vi "setLockin_phi.vi"(8 "error in (no error)":errorcluster, 9 "new phi (deg)":dbl, 10 "lockin Channel":i32, 11 "Channels: Lockin":T1={"REF f (Hz)"=[13.0], "REF phi (deg)"=[0.0]} {"REF phi (deg)" format="%#_3g"}) -> (0 "error out":errorcluster, 3 "Channels: Lockin":T1={"REF f (Hz)"=[13.0], "REF phi (deg)"=[0.0]} {"REF phi (deg)" format="%#_3g"})   [LabVIEW 2016]
uses:
  Typedefs/REF-cluster.ctl
  Typedefs/REF_f-array.ctl
  Typedefs/REF_phi-array.ctl
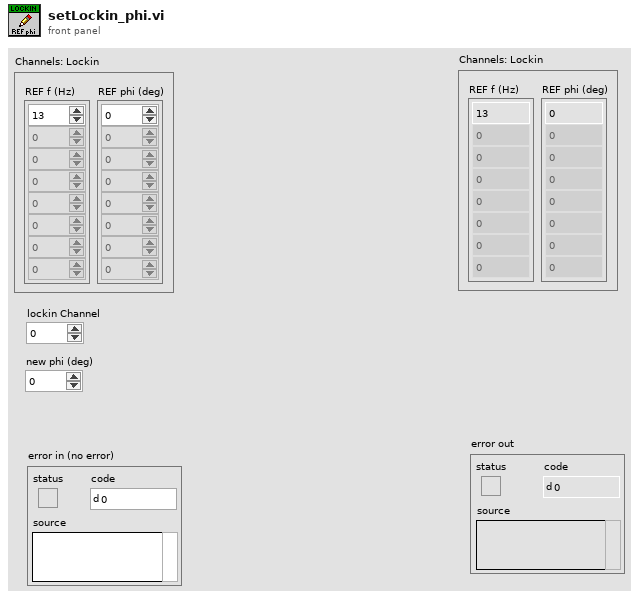
[diagram p1: front panel]
types:
  T1 = typedef "REF-cluster.ctl" = cluster{"REF f (Hz)":T2, "REF phi (deg)":T3}
  T2 = typedef "REF_f-array.ctl" = dbl[]
  T3 = typedef "REF_phi-array.ctl" = dbl[]
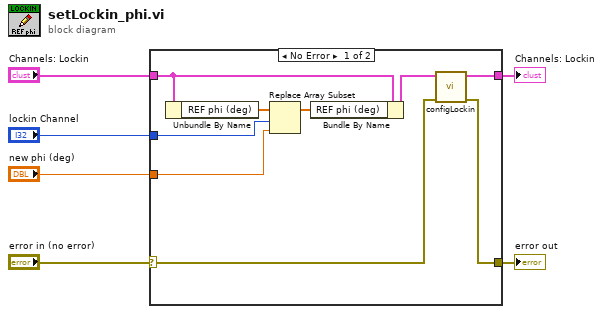
[diagram p0: block diagram]
diagram:
  n1 = case shown="No Error" "error in (no error)" {
    selector: "error in (no error)" -> [w8 w17]
    tunnel: "Channels: Lockin" -> [w13 w16]
    tunnel: [w9 w16] -> w5
    tunnel: "lockin Channel" -> [w12 _]
    tunnel: "new phi (deg)" -> [w11 _]
    tunnel: [w7 w17] -> w1
    frame No Error {
      n2 = Unbundle By Name(w13) -> ("REF phi (deg)"=w14:T3)
      n3 = Replace Array Subset(array=w14, new element=w11, index=w12) -> (w15:T3)
      n4 = Bundle By Name(cluster=w13, "REF phi (deg)"=w15) -> (w10:T1)
      n5 = call "configLockin.vi"("error in (no error)"=w8, "Channels: Lockin in"=w10) -> ("error out"=w7:errorcluster, "Channels: Lockin out"=w9:T1)  [unwired: 8 in]
    }
    frame Error {
    }
  }
  "Channels: Lockin" <- w5
  "error out" <- w1
